vi "G_Horno.vi"() -> ()   [LabVIEW 2020]
panel:
  out "Horno":T1 {"Termometro" scale=0.0..200.0}
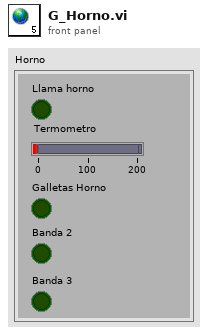
[diagram p1: front panel]
types:
  T1 = cluster{"Llama horno":bool, "Termometro":dbl, "Galletas Horno":bool, "Banda 2":bool, "Banda 3":bool}
diagram:
